vi "setAverage.vi"(8 "error in (no error)":errorcluster, 9 "Average Factor":i32, 10 "Average?":enum16{"ON", "OFF"}(ring), 11 "Instrument.VSource in":refnum<class "Instrument.VNA.lvclass">) -> (0 "error out":errorcluster, 3 "Instrument.VSource out":refnum<class "Instrument.VNA.lvclass">)   [LabVIEW 2019, in "Instrument.VNA.lvclass"]
uses:
  Instrument.VNA.lvclass
  C:/Users/patrick/Documents/GitHub/Instrument-Framework/lvsrc/Instrument/Instrument.lvclass
  Typedefs/setAverage--cluster.ctl
  a7778a3f-2d83-487d-a440-3f810fbb8fcf.vi
  a7778a3f-2d83-487d-a440-3f810fbb8fcf.vi/bd4f0d91-abba-4def-b7ab-654ced9db6e8.vi
  a7778a3f-2d83-487d-a440-3f810fbb8fcf.vi/bd4f0d91-abba-4def-b7ab-654ced9db6e8.vi/3f1acf57-bfa2-4086-ba1d-0ec87a72f942.vi
  a7778a3f-2d83-487d-a440-3f810fbb8fcf.vi/bd4f0d91-abba-4def-b7ab-654ced9db6e8.vi/634d2af2-d5e9-4a33-822d-ba37270a580a.vi
  Instrument/Private/Get RC Connection Status.vi
  Instrument/API/Send and Receive.vi
  <vilib>/Utility/Data Type/Get Type Information.vi
  <vilib>/JDP Science/JSONtext/JSON text to Variant.vi
  <vilib>/JDP Science/JSONtext/LVClass Serializer/JSONtext LVClass Serializer.lvclass
  Instrument/Instrument.lvclass
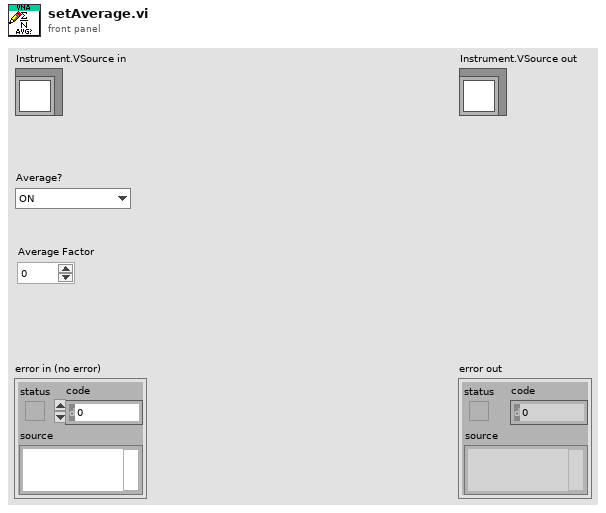
[diagram p1: front panel]
types:
  T1 = typedef "Instrument.VNA.lvclass/setAverage--cluster.ctl" = cluster{"average":enum16{"ON", "OFF"}, "factor":i32}
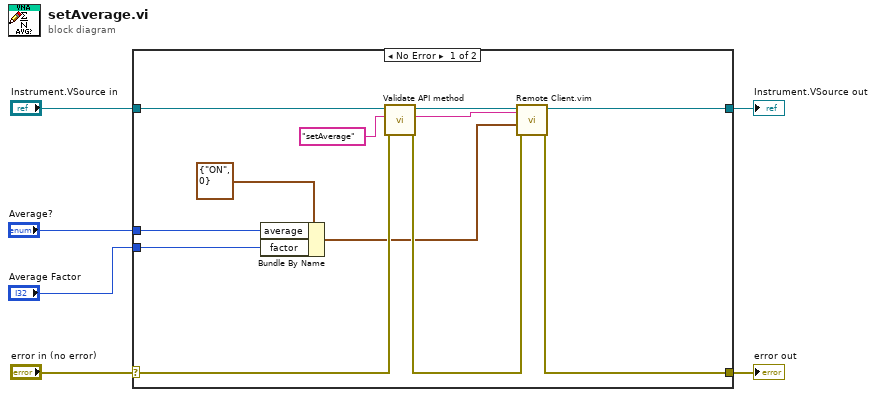
[diagram p0: block diagram]
diagram:
  n1 = case shown="No Error" "error in (no error)" {
    selector: "error in (no error)" -> [w13 w20]
    tunnel: [w12 w20] -> w5
    tunnel: [w14 w19] -> w3
    tunnel: "Instrument.VSource in" -> [w15 w19]
    tunnel: "Average Factor" -> [w9 _]
    tunnel: "Average?" -> [w8 _]
    frame No Error {
      n2 = Bundle By Name(cluster=T1 {"average"=enum."ON", "factor"=0} ("setAverage"), "average"=w8, "factor"=w9) -> (w7:T1)
      n3 = call "Validate API method.vi"("error in (no error)"=w13, "Command in"="setAverage" ("error message (\"\")"), "Instrument in"=w15) -> ("error out"=w11:errorcluster, "command out"=w17:string, "Instrument out"=w16:refnum<class "Instrument.VNA.lvclass">)  [unwired: 6 in]
      n4 = call "Remote Client.vim"("Data Out type"=w17, "error in (no error)"=w11, "Data in"=w7, "Instrument in"=w16) -> ("error out"=w12:errorcluster, "Instrument out"=w14:refnum<class "Instrument.VNA.lvclass">)  [unwired: 4 in, 2 out]
    }
    frame Error {
    }
  }
  "error out" <- w5
  "Instrument.VSource out" <- w3
